vi "VI-Add XControl File.vi"(0 "XCtl Path in":path=path "C:/Users/hancock/Desktop/Test/Test.xctl", 2 "Add to folder":string="Methods", 5 "Template":path=path "C:/Users/hancock/Desktop/Test/Test.xctl", 9 "Name":string, 11 "error in (no error)":errorcluster) -> (4 "XCtl Path out":path=path "C:/Users/hancock/Desktop/Test/Test.xctl", 8 "local path":path, 15 "error out":errorcluster)   [LabVIEW 2015]
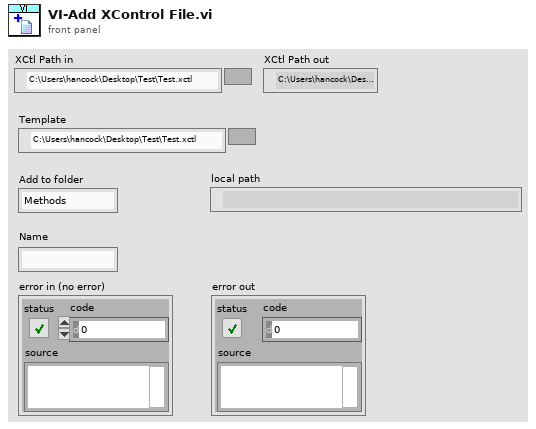
[diagram p1: front panel]
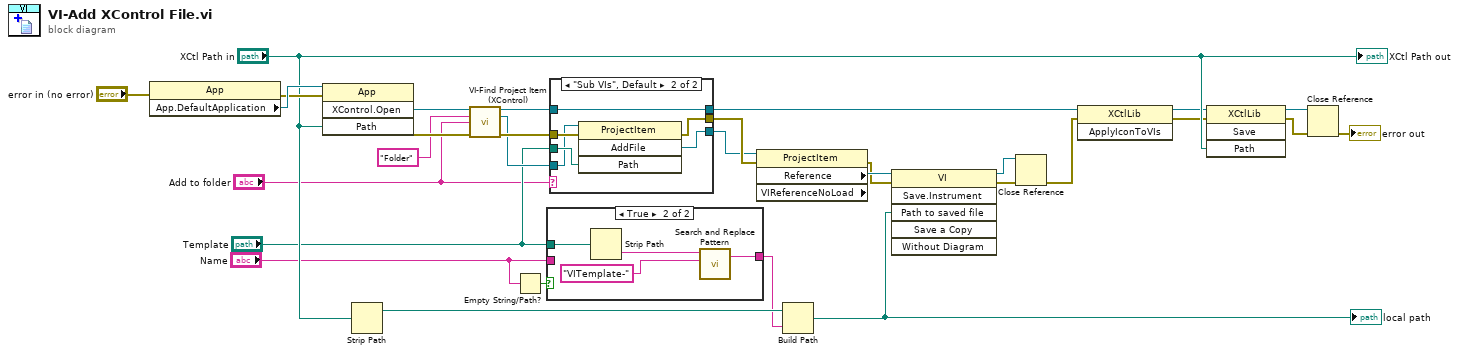
[diagram p0: block diagram]
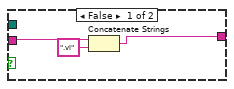
[diagram p2: hidden frame]
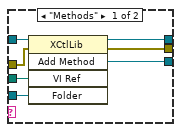
[diagram p3: hidden frame]
diagram:
  n1 = property class="App"(error in="error in (no error)") -> (error out=w25:errorcluster, "App.DefaultApplication"=w26:refnum<vi>)  [unwired: 1 in, 1 out]
  n2 = invoke class="App" method="XControl.Open"(reference=w26, error in=w25, "Path"="XCtl Path in") -> (error out=w28:errorcluster, "Open XControl"=w29:refnum<vi>)  [unwired: 1 in, 2 out]
  n3 = Strip Path(path="XCtl Path in") -> (stripped path=w27:path)  [unwired: 1 out]
  n4 = call "VI-Find Project Item (XControl).vi"("XCtlLib Refnum"=w29, "Type"="Folder" ("y"), "Name"="Add to folder", "error in (no error)"=w28) -> ("reference out"=w24:refnum<vi>, "ProjectItem"=w19:refnum<vi>, "error out"=w21:errorcluster)  [unwired: 9 in]
  n5 = Empty String/Path?(string/path="Name") -> (empty?=w5:bool)
  n6 = case shown="True" w5 {
    tunnel: "Template" -> [_ w37]
    tunnel: [w31 w34] -> w10
    tunnel: "Name" -> [w33 _]
    frame False {
      n7 = Concatenate Strings(w33, ".vi" ("string")) -> (w31:string)
    }
    frame True {
      n8 = Strip Path(path=w37) -> (name=w36:string)  [unwired: 1 out]
      n9 = call <vilib>:"Search and Replace Pattern.vi"("string"=w36, "regular expression (\"\")"="VITemplate-" ("regular expression (\"\")")) -> ("result string"=w34:string)  [unwired: 3 in, 1 out]
    }
  }
  n10 = case shown="\"Sub VIs\", Default" "Add to folder" {
    tunnel: w24 -> [w44 w45]
    tunnel: w21 -> [w43 w50]
    tunnel: [w42 w49] -> w20
    tunnel: w19 -> [w41 w46]
    tunnel: [w40 w48] -> w18
    tunnel: "Template" -> [w39 w47]
    tunnel: [w38 w45] -> w4
    frame "Methods" {
      n11 = invoke class="XCtlLib" method="Add Method"(reference=w44, error in=w43, "VI Ref"=w39, "Folder"=w41) -> (reference out=w38:refnum<vi>, error out=w42:errorcluster, "Add Method"=w40:refnum<vi>)  [unwired: 1 in, 2 out]
    }
    frame "Sub VIs", Default {
      n12 = invoke class="ProjectItem" method="AddFile"(reference=w46, error in=w50, "Path"=w47) -> (error out=w49:errorcluster, "AddFile"=w48:refnum<vi>)  [unwired: 1 in, 2 out]
    }
  }
  n13 = property class="ProjectItem" props=["Reference", "VIReferenceNoLoad"](reference=w18, error in=w20) -> (error out=w12:errorcluster, "Reference"=w13:refnum<vi>)  [unwired: 2 out]
  n14 = Build Path(base path=w27, name or relative path=w10) -> (appended path=w16:path)
  "local path" <- w16
  n15 = invoke class="VI" method="Save.Instrument"(reference=w13, error in=w12, "Path to saved file"=w16) -> (reference out=w7:refnum<vi>, error out=w8:errorcluster)  [unwired: 3 in, 4 out]
  n16 = Close Reference(reference=w7, error in (no error)=w8) -> (error out=w3:errorcluster)
  n17 = invoke class="XCtlLib" method="ApplyIconToVIs"(reference=w4, error in=w3) -> (reference out=w1:refnum<vi>, error out=w2:errorcluster)  [unwired: 1 in, 1 out]
  n18 = invoke class="XCtlLib" method="Save"(reference=w1, error in=w2, "Path"="XCtl Path in") -> (reference out=w17:refnum<vi>, error out=w15:errorcluster)  [unwired: 1 in, 2 out]
  n19 = Close Reference(reference=w17, error in (no error)=w15) -> (error out=→"error out":errorcluster)
  "XCtl Path out" <- "XCtl Path in"
